vi "Kugel V9.vi"() -> ()   [LabVIEW 2020]
doc: "Illustrates the different data types that can be wired to the Case Selector terminal of a Case Structure. A Case Selector terminal can accept one of five possible data types: Boolean, error cluster, integer, enum, or string."
uses:
  Program Files (x86)/National Instruments/LabVIEW 2020/examples/Structures/Case Structure/support/Case Structure - Enum Options.ctl
  <vilib>/Utility/error.llb/DialogType.ctl
  <vilib>/DAQmx/write.llb/DAQmx Write (Digital Bool 1Line 1Point).vi
  <vilib>/DAQmx/read.llb/DAQmx Read (Analog DBL 1Chan 1Samp).vi
  <vilib>/Analysis/baseanly.llb/Mean (DBL).vi
  <vilib>/DAQmx/read.llb/DAQmx Read (Analog Wfm 1Chan NSamp).vi
  <vilib>/DAQmx/read.llb/DAQmx Read (Analog 1D Wfm NChan NSamp).vi
  <vilib>/DAQmx/create/channels.llb/DAQmx Create Channel (DO-Digital Output).vi
  <vilib>/DAQmx/create/channels.llb/DAQmx Create Channel (AI-Voltage-Basic).vi
  <vilib>/DAQmx/configure/timing.llb/DAQmx Timing (Sample Clock).vi
  <vilib>/DAQmx/miscellaneous.llb/DAQmx Fill In Error Info.vi
  <vilib>/DAQmx/configure/task.llb/DAQmx Configure Logging (TDMS).vi
  <vilib>/Waveform/WDTOps.llb/WDT Index Channel DBL.vi
  <vilib>/Analysis/NI_AALBase.lvlib
panel:
  out "P-Ex3 Max ungefilter":dbl caption="bar (max)" format="%0.2f"
  out "P-Ex3 Max gefilter":dbl caption="bar (max)" format="%0.2f"
  out "Current Save Path":path
  in  "User":string="unknown"
  in  "Serie":i32=1
  in  "Gas in Vol-%":dbl format="%.1f"
  in  "Gas":string(combo)="NoGas"
  in  "Weight [g]":dbl format="%.1f"
  in  "Dust":string(combo)="NoDust"
  out "Waveform Graph Staub":waveform(dbl)(graph)
  out "Pressure in V":dbl format="%0.3f"
  out "P-Ex3":dynamicdata(graph)
  out "P-Ex1":dynamicdata(graph)
  out "gemessene Spannungen":waveform(dbl)[](graph)
  in  "Ignition":bool
  in  "IN":bool
  in  "Reset":bool
  in  "OUT":bool
  in  "stop":bool
  out "Pressure in bar":dbl format="%0.3f"
  out "Pressure in bar":dbl(knob) scale=0.0..22.0
  in  "Option 1: manual operation\nOption 2: Ignition":T1
  # "Option 1"
  # "Option 2"
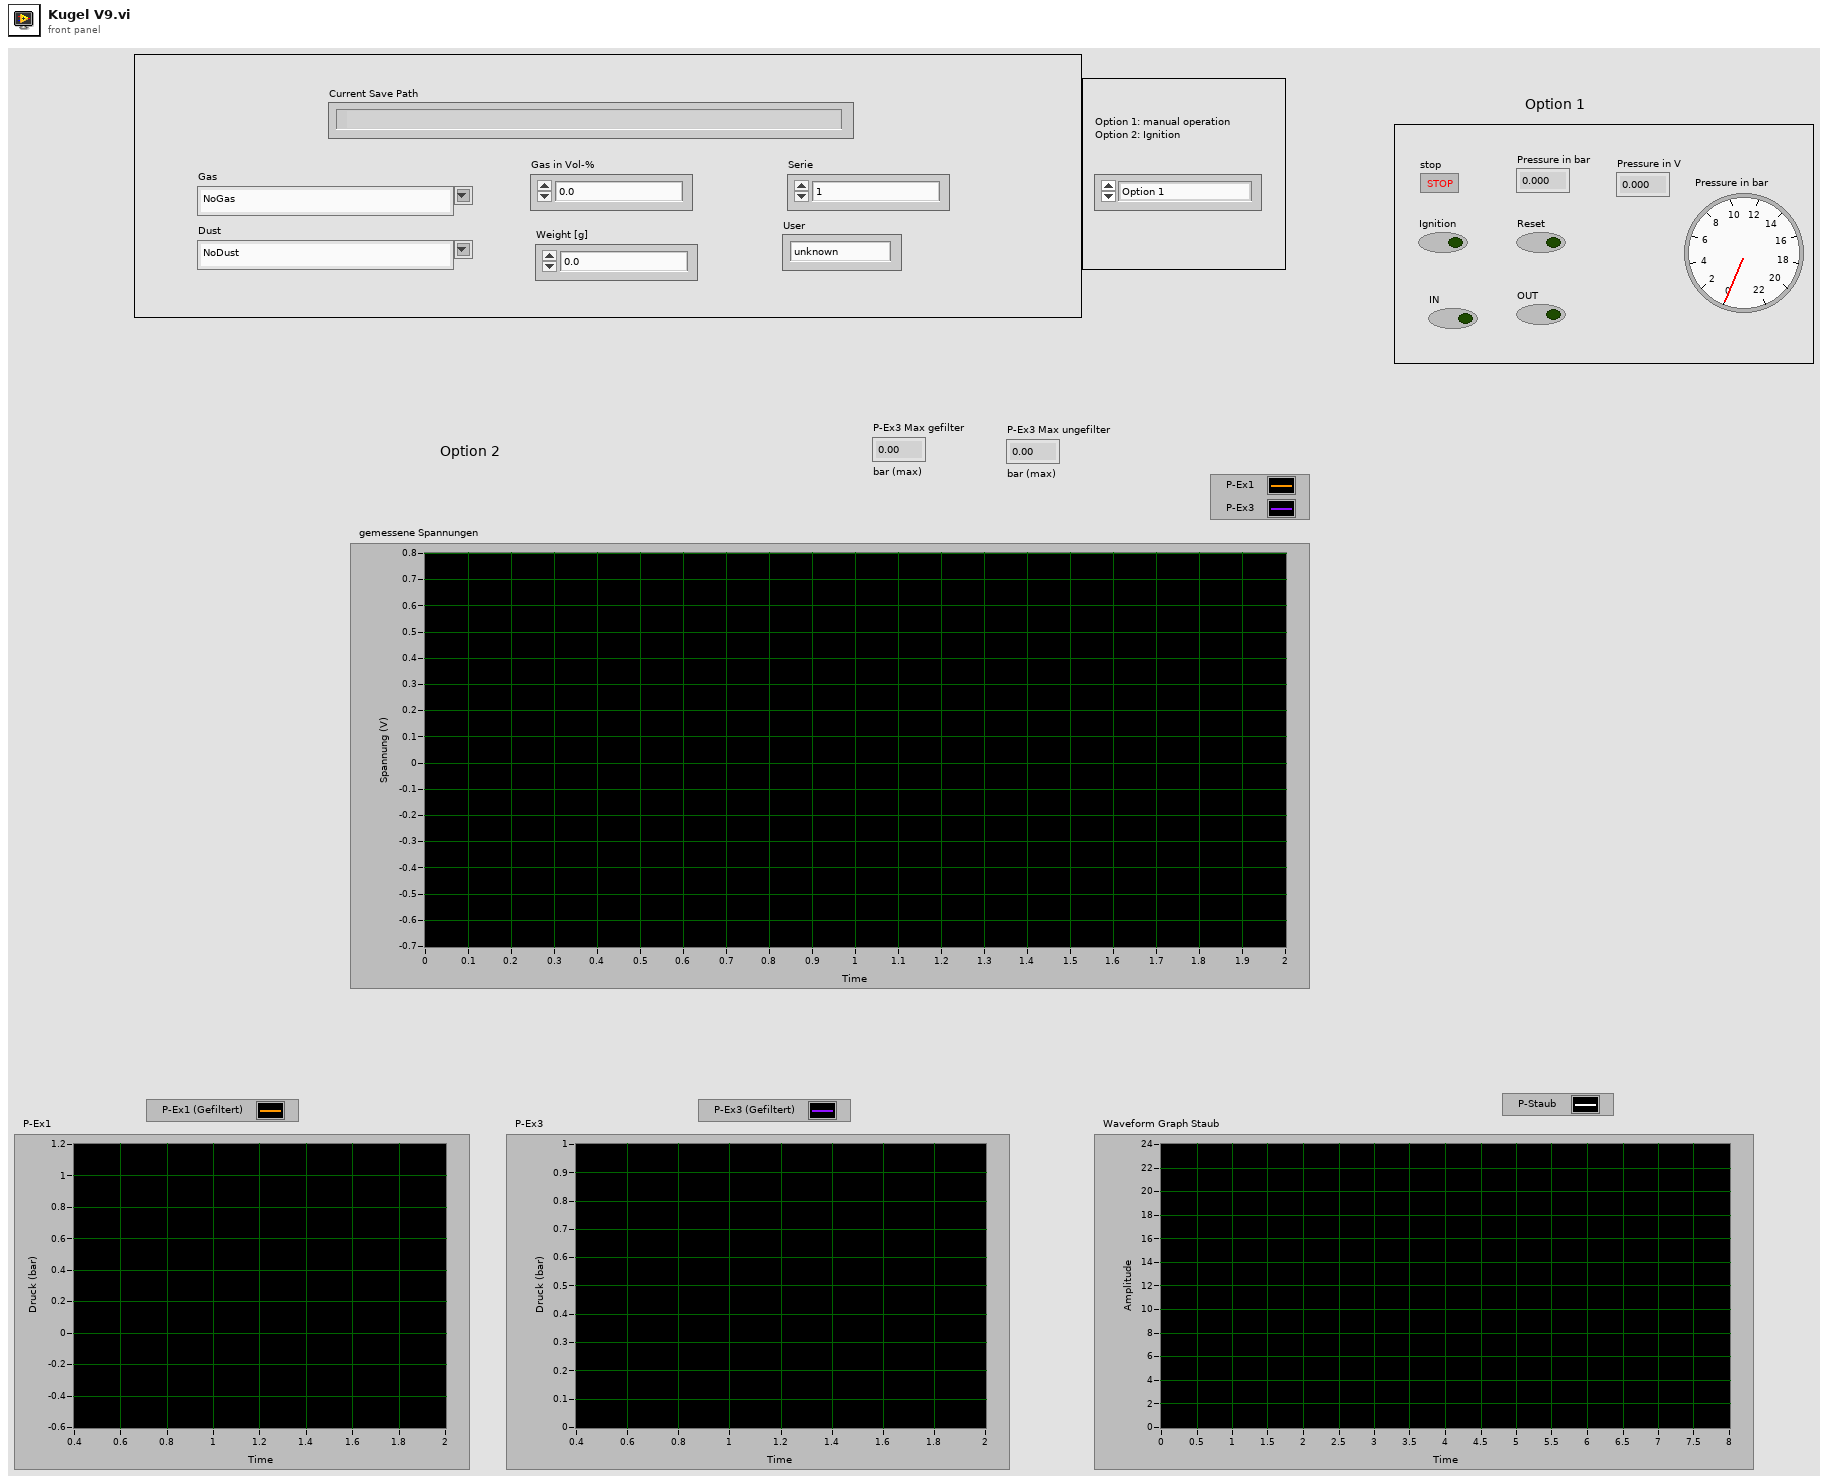
[diagram p1: front panel]
types:
  T1 = typedef "Case Structure - Enum Options.ctl" = enum16{"Option 1", "Option 2", "Option 3", "Option 4", "Option 5"}
  T2 = typedef "DialogType.ctl" = u16
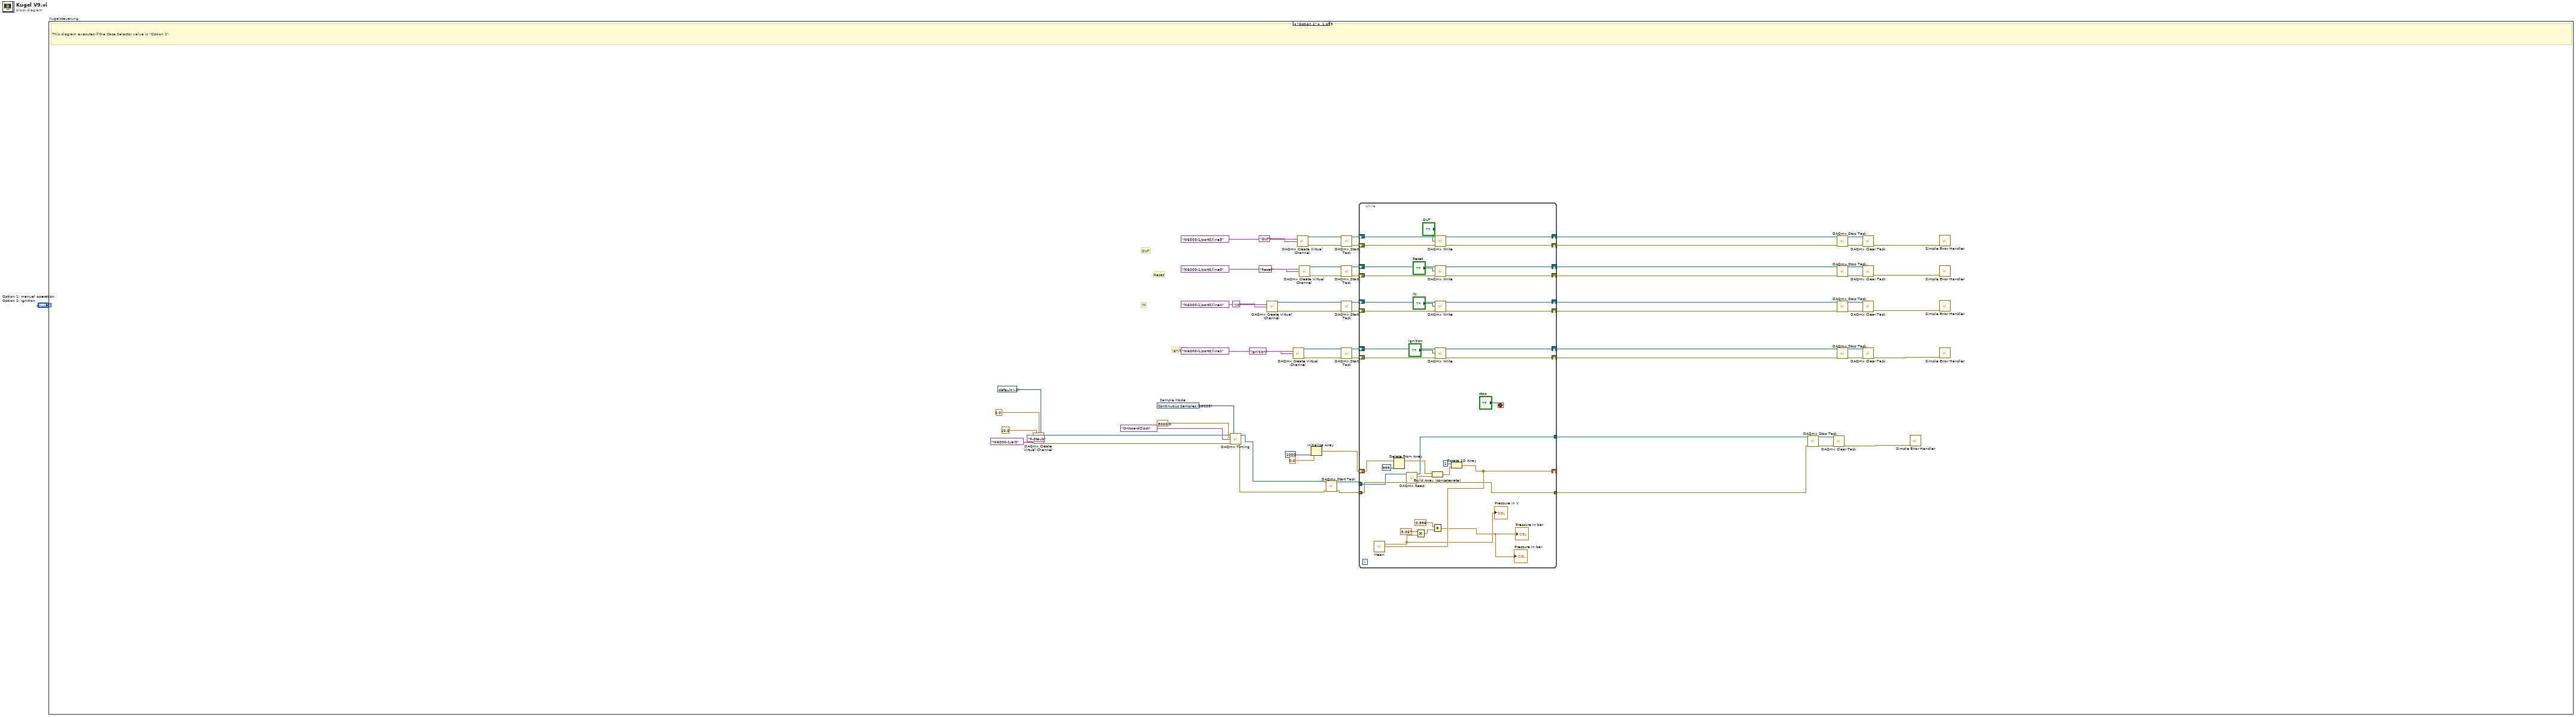
[diagram p0: block diagram]
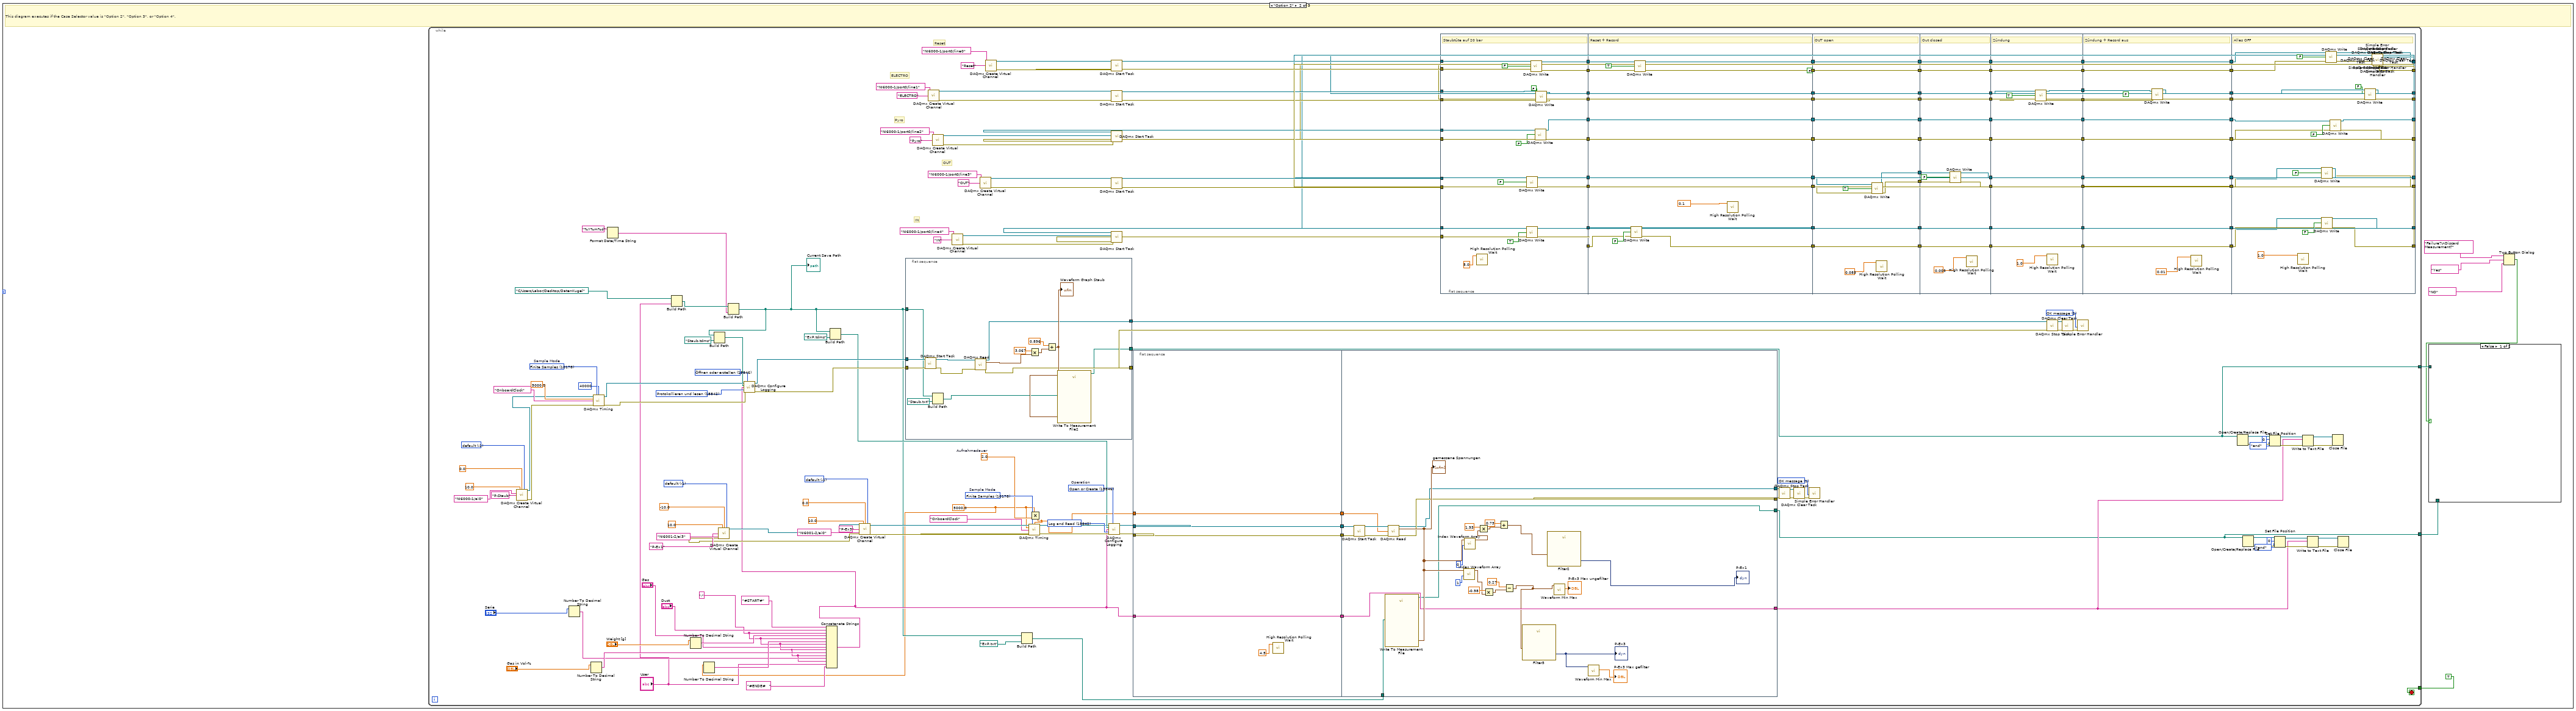
[diagram p2: hidden frame]
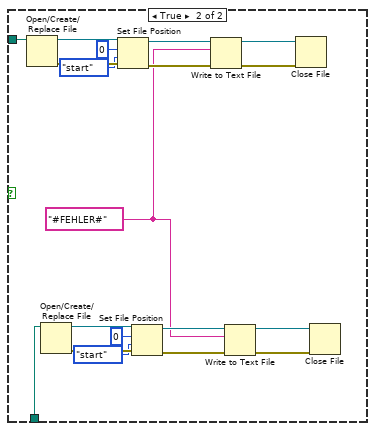
[diagram p3: hidden frame]
diagram:
  n1 = case "Kugelsteuerung" shown="\"Option 1\"" "Option 1: manual operation\nOption 2: Ignition" {
    frame "Option 1" {
      w19 = -1 items=["default"=-1, "RSE"=10083, "NRSE"=10078, "Differential"=10106, "Pseudodifferential"=12529] ("Terminal Configuration")
      w23 = 10123 items=["Finite Samples"=10178, "Continuous Samples"=10123, "Hardware Timed Single Point"=12522]  # Sample Mode
      # "Ignition"
      # "IN"
      # "OUT"
      # "Reset"
      # "This diagram executes if the Case Selector value is \"Option 1\"."
      n2 = call-poly <vilib>:"DAQmx Create Virtual Channel.vi"("maximum value"=10.0 ("Max Voltage P-Ex3"), "minimum value"=0.0 ("Min Voltage P-Ex3"), "input terminal configuration"=w19, "physical channels"=tag "NI6000-1/ai0" ("Physical Channel"), "name to assign"="P-Staub") -> ("task out"=w21:refnum<k21>, "error out"=w22:errorcluster)  [unwired: 9 in]
      n3 = call-poly <vilib>:"DAQmx Timing.vi"("task/channels in"=w21, "sample mode"=w23, "rate"=5000.0 ("Sample Rate"), "source"=tag "OnboardClock" ("Sample Clock Source"), "error in"=w22) -> ("task out"=w6:refnum<k21>, "error out"=w5:errorcluster)  [unwired: 9 in]
      n4 = call-poly <vilib>:"DAQmx Create Virtual Channel.vi"("lines"=tag "NI6000-1/port0/line4", "name to assign"="IN") -> ("task out"=w54:refnum<k21>, "error out"=w53:errorcluster)  [unwired: 12 in]
      n5 = call-poly <vilib>:"DAQmx Create Virtual Channel.vi"("lines"=tag "NI6000-1/port0/line1", "name to assign"="Ignition") -> ("task out"=w51:refnum<k21>, "error out"=w50:errorcluster)  [unwired: 12 in]
      n6 = call-poly <vilib>:"DAQmx Create Virtual Channel.vi"("lines"=tag "NI6000-1/port0/line3", "name to assign"="OUT") -> ("task out"=w57:refnum<k21>, "error out"=w56:errorcluster)  [unwired: 12 in]
      n7 = call-poly <vilib>:"DAQmx Create Virtual Channel.vi"("lines"=tag "NI6000-1/port0/line0", "name to assign"="Reset") -> ("task out"=w67:refnum<k21>, "error out"=w66:errorcluster)  [unwired: 12 in]
      n8 = Initialize Array(0.0 ("element"), 1000 ("dimension size")) -> (w4:dbl[])
      n9 = call <vilib>:"DAQmx Start Task.vi"("task/channels in"=w6, "error in"=w5) -> ("task out"=w8:refnum<k21>, "error out"=w7:errorcluster)  [unwired: 12 in]
      n10 = call <vilib>:"DAQmx Start Task.vi"("task/channels in"=w57, "error in"=w56) -> ("task out"=w29:refnum<k21>, "error out"=w28:errorcluster)  [unwired: 12 in]
      n11 = call <vilib>:"DAQmx Start Task.vi"("task/channels in"=w67, "error in"=w66) -> ("task out"=w31:refnum<k21>, "error out"=w30:errorcluster)  [unwired: 12 in]
      n12 = call <vilib>:"DAQmx Start Task.vi"("task/channels in"=w54, "error in"=w53) -> ("task out"=w25:refnum<k21>, "error out"=w24:errorcluster)  [unwired: 12 in]
      n13 = call <vilib>:"DAQmx Start Task.vi"("task/channels in"=w51, "error in"=w50) -> ("task out"=w27:refnum<k21>, "error out"=w26:errorcluster)  [unwired: 12 in]
      n14 = while {
        shift-right: [w104] -> w39
        shift-left: w31 -> [w96]
        shift-right: [w103] -> w38
        shift-left: w30 -> [w95]
        shift-right: [w102] -> w37
        shift-left: w29 -> [w94]
        shift-right: [w101] -> w36
        shift-left: w28 -> [w93]
        shift-right: [w100] -> w35
        shift-left: w27 -> [w92]
        shift-right: [w99] -> w34
        shift-left: w26 -> [w91]
        shift-right: [w98] -> w33
        shift-left: w25 -> [w90]
        shift-right: [w97] -> w32
        shift-left: w24 -> [w89]
        tunnel: w8 -> [w83]
        tunnel: w7 -> [w82]
        tunnel: [w81] -> w11
        tunnel: [w80] -> w10
        shift-right: [w74] -> _
        shift-left: w4 -> [w78]
        stop <- "stop" stop-if-true
        n15 = Delete From Array(array=w78, index=999) -> (array with subset deleted=w77:dbl[])  [unwired: 1 in, 1 out]
        n16 = call-poly <vilib>:"DAQmx Read.vi"("task/channels in"=w83, "error in"=w82) -> ("task out"=w81:refnum<k21>, "data"=w79:dbl, "error out"=w80:errorcluster)  [unwired: 11 in]
        n17 = Build Array (concatenate)(w77, w79) -> (w75:dbl[])
        n18 = call-poly <vilib>:"DAQmx Write.vi"("task/channels in"=w94, "data"="OUT", "error in"=w93) -> ("task out"=w102:refnum<k21>, "error out"=w101:errorcluster)  [unwired: 10 in, 1 out]
        n19 = call-poly <vilib>:"DAQmx Write.vi"("task/channels in"=w96, "data"="Reset", "error in"=w95) -> ("task out"=w104:refnum<k21>, "error out"=w103:errorcluster)  [unwired: 10 in, 1 out]
        n20 = call-poly <vilib>:"DAQmx Write.vi"("task/channels in"=w90, "data"="IN", "error in"=w89) -> ("task out"=w98:refnum<k21>, "error out"=w97:errorcluster)  [unwired: 10 in, 1 out]
        n21 = call-poly <vilib>:"DAQmx Write.vi"("task/channels in"=w92, "data"="Ignition", "error in"=w91) -> ("task out"=w100:refnum<k21>, "error out"=w99:errorcluster)  [unwired: 10 in, 1 out]
        n22 = Rotate 1D Array(1:w75, 2:1 ("n")) -> (0:w74:dbl[])
        n23 = call-poly <vilib>:"Mean.vi"("X"=w74) -> ("mean"=w68:dbl)  [unwired: 1 out]
        "Pressure in V" <- w68
        n24 = Multiply(x=3.067, y=w68) -> (x*y=w72:dbl)
        n25 = Add(x=0.896 ("y"), y=w72) -> (x+y=→"Pressure in bar" →"Pressure in bar":dbl)
      }
      n26 = call <vilib>:"DAQmx Stop Task.vi"("task/channels in"=w11, "error in"=w10) -> ("task out"=w14:refnum<k21>, "error out"=w13:errorcluster)  [unwired: 12 in]
      n27 = call <vilib>:"DAQmx Clear Task.vi"("task in"=w14, "error in"=w13) -> ("error out"=w12:errorcluster)  [unwired: 13 in]
      n28 = call <vilib>:"DAQmx Stop Task.vi"("task/channels in"=w37, "error in"=w36) -> ("task out"=w61:refnum<k21>, "error out"=w60:errorcluster)  [unwired: 12 in]
      n29 = call <vilib>:"DAQmx Stop Task.vi"("task/channels in"=w39, "error in"=w38) -> ("task out"=w65:refnum<k21>, "error out"=w64:errorcluster)  [unwired: 12 in]
      n30 = call <vilib>:"DAQmx Stop Task.vi"("task/channels in"=w33, "error in"=w32) -> ("task out"=w46:refnum<k21>, "error out"=w45:errorcluster)  [unwired: 12 in]
      n31 = call <vilib>:"DAQmx Stop Task.vi"("task/channels in"=w35, "error in"=w34) -> ("task out"=w49:refnum<k21>, "error out"=w48:errorcluster)  [unwired: 12 in]
      n32 = call <vilib>:"DAQmx Clear Task.vi"("task in"=w61, "error in"=w60) -> ("error out"=w59:errorcluster)  [unwired: 13 in]
      n33 = call <vilib>:"DAQmx Clear Task.vi"("task in"=w65, "error in"=w64) -> ("error out"=w63:errorcluster)  [unwired: 13 in]
      n34 = call <vilib>:"DAQmx Clear Task.vi"("task in"=w46, "error in"=w45) -> ("error out"=w44:errorcluster)  [unwired: 13 in]
      n35 = call <vilib>:"DAQmx Clear Task.vi"("task in"=w49, "error in"=w48) -> ("error out"=w47:errorcluster)  [unwired: 13 in]
      n36 = call <vilib>:"Simple Error Handler.vi"("error in (no error)"=w12) -> ()  [unwired: 4 in, 5 out]
      n37 = call <vilib>:"Simple Error Handler.vi"("error in (no error)"=w59) -> ()  [unwired: 4 in, 5 out]
      n38 = call <vilib>:"Simple Error Handler.vi"("error in (no error)"=w63) -> ()  [unwired: 4 in, 5 out]
      n39 = call <vilib>:"Simple Error Handler.vi"("error in (no error)"=w44) -> ()  [unwired: 4 in, 5 out]
      n40 = call <vilib>:"Simple Error Handler.vi"("error in (no error)"=w47) -> ()  [unwired: 4 in, 5 out]
    }
    frame "Option 2" {
      # "This diagram executes if the Case Selector value is \"Option 2\", \"Option 3\", or \"Option 4\"."
      n41 = while {
        tunnel: TRUE ("Stopp-Schaltfläche") -> [w201]
        tunnel: [w145] -> w110
        tunnel: [w144] -> w109
        stop <- w201 stop-if-true
        w131 = 5000.0 ("Sample Rate")
        w165 = ";" ("String")
        w180 = 15846 items=["Öffnen"=10437, "Öffnen oder erstellen"=15846, "Erstellen oder ersetzen"=15847, "Erstellen"=15848] ("operation")
        w181 = 15842 items=["Aus"=10231, "Protokoll"=15844, "Protokollieren und lesen"=15842] ("logging mode")
        w189 = -1 items=["default"=-1, "RSE"=10083, "NRSE"=10078, "Differential"=10106, "Pseudodifferential"=12529] ("Terminal Configuration")
        w194 = 10178 items=["Finite Samples"=10178, "Continuous Samples"=10123, "Hardware Timed Single Point"=12522]  # Sample Mode
        w197 = T2 1 items=["no dialog", "OK message", "continue or stop message", "OK message + warnings", "continue/stop + warnings"] ("type of dialog (OK msg:1)")
        w208 = 2.0  # Aufnahmedauer
        w210 = T2 1 items=["no dialog", "OK message", "continue or stop message", "OK message + warnings", "continue/stop + warnings"] ("type of dialog (OK msg:1)")
        w226 = 15842 items=["Off"=10231, "Log and Read"=15842] ("Logging Mode")
        w224 = -1 items=["default"=-1, "RSE"=10083, "NRSE"=10078, "Differential"=10106, "Pseudodifferential"=12529] ("Terminal Configuration")
        w216 = -1 items=["default"=-1, "RSE"=10083, "NRSE"=10078, "Differential"=10106, "Pseudodifferential"=12529] ("Terminal Configuration 3")
        w227 = 15846 items=["Open"=10437, "Open or Create"=15846, "Create or Replace"=15847, "Create"=15848]  # Operation
        w230 = 10178 items=["Finite Samples"=10178, "Continuous Samples"=10123, "Hardware Timed Single Point"=12522]  # Sample Mode
        # "ELECTRO"
        # "Pyro"
        # "IN"
        # "OUT"
        # "Reset"
        n42 = call-poly <vilib>:"DAQmx Create Virtual Channel.vi"("maximum value"=10.0 ("Max Voltage P-Ex3"), "minimum value"=0.0 ("Min Voltage P-Ex3"), "input terminal configuration"=w189, "physical channels"=tag "NI6000-1/ai0" ("Physical Channel"), "name to assign"="P-Staub") -> ("task out"=w185:refnum<k21>, "error out"=w186:errorcluster)  [unwired: 9 in]
        n43 = Number To Decimal String(number="Serie") -> (decimal integer string=w166:string)  [unwired: 1 in]
        n44 = Number To Decimal String(number="Gas in Vol-%") -> (decimal integer string=w168:string)  [unwired: 1 in]
        n45 = call-poly <vilib>:"DAQmx Timing.vi"("task/channels in"=w185, "sample mode"=w194, "samples per channel"=40000, "rate"=5000.0 ("Sample Rate"), "source"=tag "OnboardClock" ("Sample Clock Source"), "error in"=w186) -> ("task out"=w183:refnum<k21>, "error out"=w182:errorcluster)  [unwired: 8 in]
        n46 = Format Date/Time String(time format string (%c)="%Y%m%d" ("Zeitformatierungs-String (%c)")) -> (date/time string=w140:string)  [unwired: 2 in]
        n47 = Build Path(base path=path "C:/Users/Labor/Desktop/DatenKugel" ("Choose Path"), name or relative path="User") -> (appended path=w142:path)
        n48 = Number To Decimal String(number="Weight [g]") -> (decimal integer string=w173:string)  [unwired: 1 in]
        n49 = Number To Decimal String(number=w131) -> (decimal integer string=w171:string)  [unwired: 1 in]
        n50 = call-poly <vilib>:"DAQmx Create Virtual Channel.vi"("maximum value"=10.0 ("Max Voltage P-Ex1"), "minimum value"=-10.0 ("Min Voltage P-Ex1"), "input terminal configuration"=w216, "physical channels"=tag "NI6001-2/ai3" ("Physical Channel 3"), "name to assign"="P-Ex1") -> ("task out"=w203:refnum<k21>, "error out"=w202:errorcluster)  [unwired: 9 in]
        n51 = Build Path(base path=w142, name or relative path=w140) -> (appended path=w133:path)
        "Current Save Path" <- w133
        n52 = Build Path(base path=w133, name or relative path=path "Staub.tdms" ("Name oder relativer Pfad")) -> (appended path=w138:path)
        n53 = Concatenate Strings("#START#" ("String"), "Dust", w165, w173, w165, w171, w165, "Gas", w165, w168, w165, w166, w165, "User", "#ENDE#   " ("String")) -> (w175:string)
        n54 = call-poly <vilib>:"DAQmx Configure Logging.vi"("task/channels in"=w183, "operation"=w180, "file path"=w138, "group name"=w175, "logging mode"=w181, "error in"=w182) -> ("task out"=w179:refnum<k21>, "error out"=w178:errorcluster)  [unwired: 8 in]
        n55 = Build Path(base path=w133, name or relative path=path "ExP.tdms" ("Name oder relativer Pfad")) -> (appended path=w134:path)
        n56 = call-poly <vilib>:"DAQmx Create Virtual Channel.vi"("task in"=w203, "maximum value"=10.0 ("Max Voltage P-Ex3"), "minimum value"=0.0 ("Min Voltage P-Ex3"), "input terminal configuration"=w224, "physical channels"=tag "NI6001-2/ai0" ("Physical Channel"), "name to assign"="P-Ex3", "error in"=w202) -> ("task out"=w228:refnum<k21>, "error out"=w229:errorcluster)  [unwired: 7 in]
        n57 = flat-sequence {
          tunnel: w179 -> [w359]
          tunnel: w178 -> [w358]
          tunnel: [w354] -> w177
          tunnel: [w353] -> w176
          tunnel: [w352] -> w145
          tunnel: w133 -> [w351]
          frame #0 {
            n58 = call <vilib>:"DAQmx Start Task.vi"("task/channels in"=w359, "error in"=w358) -> ("task out"=w362:refnum<k21>, "error out"=w363:errorcluster)  [unwired: 12 in]
            n59 = Build Path(base path=w351, name or relative path=path "Staub.txt" ("Name oder relativer Pfad")) -> (appended path=w349:path)
            n60 = call-poly <vilib>:"DAQmx Read.vi"("task/channels in"=w362, "error in"=w363) -> ("task out"=w354:refnum<k21>, "data"=w361:waveform(dbl), "error out"=w353:errorcluster)  [unwired: 11 in]
            n61 = Multiply(x=3.067, y=w361) -> (x*y=w360:waveform(dbl))
            n62 = Add(x=0.896 ("y"), y=w360) -> (x+y=w355:waveform(dbl))
            "Waveform Graph Staub" <- w355
            n63 = call "Write To Measurement File2"("Signals"=w355, "Filename"=w349) -> ("Filename Out"=w352:path)  [unwired: 15 in, 2 out]
          }
        }
        n64 = call-poly <vilib>:"DAQmx Create Virtual Channel.vi"("lines"=tag "NI6000-1/port0/line1", "name to assign"="ELECTRO") -> ("task out"=w258:refnum<k21>, "error out"=w257:errorcluster)  [unwired: 12 in]
        n65 = call-poly <vilib>:"DAQmx Create Virtual Channel.vi"("lines"=tag "NI6000-1/port0/line2", "name to assign"="Pyro") -> ("task out"=w261:refnum<k21>, "error out"=w260:errorcluster)  [unwired: 12 in]
        n66 = call-poly <vilib>:"DAQmx Create Virtual Channel.vi"("lines"=tag "NI6000-1/port0/line4", "name to assign"="IN") -> ("task out"=w264:refnum<k21>, "error out"=w263:errorcluster)  [unwired: 12 in]
        n67 = call-poly <vilib>:"DAQmx Create Virtual Channel.vi"("lines"=tag "NI6000-1/port0/line3", "name to assign"="OUT") -> ("task out"=w271:refnum<k21>, "error out"=w269:errorcluster)  [unwired: 12 in]
        n68 = call-poly <vilib>:"DAQmx Create Virtual Channel.vi"("lines"=tag "NI6000-1/port0/line0", "name to assign"="Reset") -> ("task out"=w284:refnum<k21>, "error out"=w283:errorcluster)  [unwired: 12 in]
        n69 = Build Path(base path=w133, name or relative path=path "ExP.txt" ("Name oder relativer Pfad")) -> (appended path=w136:path)
        n70 = Multiply(x=w131, y=w208) -> (x*y=w195:dbl)
        n71 = call-poly <vilib>:"DAQmx Timing.vi"("task/channels in"=w228, "sample mode"=w230, "samples per channel"=w195, "rate"=w131, "source"=tag "OnboardClock" ("Sample Clock Source"), "error in"=w229) -> ("task out"=w220:refnum<k21>, "error out"=w219:errorcluster)  [unwired: 8 in]
        n72 = call-poly <vilib>:"DAQmx Configure Logging.vi"("task/channels in"=w220, "operation"=w227, "file path"=w134, "group name"=w175, "logging mode"=w226, "error in"=w219) -> ("task out"=w205:refnum<k21>, "error out"=w204:errorcluster)  [unwired: 8 in]
        n73 = call <vilib>:"DAQmx Start Task.vi"("task/channels in"=w284, "error in"=w283) -> ("task out"=w285:refnum<k21>, "error out"=w282:errorcluster)  [unwired: 12 in]
        n74 = call <vilib>:"DAQmx Start Task.vi"("task/channels in"=w258, "error in"=w257) -> ("task out"=w256:refnum<k21>, "error out"=w255:errorcluster)  [unwired: 12 in]
        n75 = call <vilib>:"DAQmx Start Task.vi"("task/channels in"=w261, "error in"=w260) -> ("task out"=w254:refnum<k21>, "error out"=w253:errorcluster)  [unwired: 12 in]
        n76 = call <vilib>:"DAQmx Start Task.vi"("task/channels in"=w271, "error in"=w269) -> ("task out"=w270:refnum<k21>, "error out"=w268:errorcluster)  [unwired: 12 in]
        n77 = call <vilib>:"DAQmx Start Task.vi"("task/channels in"=w264, "error in"=w263) -> ("task out"=w252:refnum<k21>, "error out"=w251:errorcluster)  [unwired: 12 in]
        n78 = flat-sequence {
          tunnel: w204 -> [w367]
          tunnel: w205 -> [w368]
          tunnel: w175 -> [w364]
          tunnel: [w364] -> w288
          tunnel: [w368] -> w287
          tunnel: [w367] -> w286
          tunnel: w195 -> [w365]
          tunnel: [w365] -> w196
          tunnel: [w378] -> w207
          tunnel: [w379] -> w206
          tunnel: w288 -> [w377]
          tunnel: w287 -> [w395]
          tunnel: w286 -> [w394]
          tunnel: w196 -> [w380]
          tunnel: [w376] -> w144
          tunnel: [w377] -> w150
          tunnel: w136 -> [w375]
          frame #0 {
            n79 = call <vilib>:"High Resolution Polling Wait.vi"("seconds to wait"=4.5 ("Staubtüte füllen")) -> ()  [unwired: 10 in, 1 out]
          }
          frame #1 {
            n80 = call <vilib>:"DAQmx Start Task.vi"("task/channels in"=w395, "error in"=w394) -> ("task out"=w392:refnum<k21>, "error out"=w393:errorcluster)  [unwired: 12 in]
            n81 = call-poly <vilib>:"DAQmx Read.vi"("task/channels in"=w392, "number of samples per channel"=w380, "error in"=w393) -> ("task out"=w378:refnum<k21>, "data"=w382:waveform(dbl)[], "error out"=w379:errorcluster)  [unwired: 10 in]
            "gemessene Spannungen" <- w382
            n82 = call "Write To Measurement File"("Signals"=w382, "Filename"=w375) -> ("Filename Out"=w376:path)  [unwired: 15 in, 2 out]
            n83 = call-poly <vilib>:"Index Waveform Array.vi"("index"=1, "waveform array"=w382) -> ("waveform"=w381:waveform(dbl))  [unwired: 8 in, 1 out]
            n84 = call-poly <vilib>:"Index Waveform Array.vi"("index"=0, "waveform array"=w382) -> ("waveform"=w383:waveform(dbl))  [unwired: 8 in, 1 out]
            n85 = Multiply(x=1.93, y=w383) -> (x*y=w385:waveform(dbl))
            n86 = Multiply(x=-0.98, y=w381) -> (x*y=w388:waveform(dbl))
            n87 = Add(x=0.73, y=w385) -> (x+y=w374:waveform(dbl))
            n88 = Subtract(x=0.27, y=w388) -> (x-y=w370:waveform(dbl))
            n89 = call "Filter3"("Signal"=w370) -> ("Filtered Signal"=w372:dynamicdata)  [unwired: 9 in, 1 out]
            "P-Ex3" <- w372
            n90 = call "Filter2"("Signal"=w374) -> ("Filtered Signal"=→"P-Ex1":dynamicdata)  [unwired: 9 in, 1 out]
            n91 = call <vilib>:"Waveform Min Max.vi"("waveform in"=w370) -> ("Y max"=→"P-Ex3 Max ungefilter":dbl)  [unwired: 5 in, 5 out]
            n92 = call <vilib>:"Waveform Min Max.vi"("waveform in"=w372) -> ("Y max"=→"P-Ex3 Max gefilter":dbl)  [unwired: 5 in, 5 out]
          }
        }
        n93 = flat-sequence {
          tunnel: w285 -> [w419]
          tunnel: w282 -> [w418]
          tunnel: w270 -> [w417]
          tunnel: w268 -> [w415]
          tunnel: w256 -> [w413]
          tunnel: w255 -> [w412]
          tunnel: w254 -> [w411]
          tunnel: w253 -> [w410]
          tunnel: w252 -> [w409]
          tunnel: w251 -> [w408]
          tunnel: [w421] -> w348
          tunnel: [w420] -> w347
          tunnel: [w416] -> w346
          tunnel: [w414] -> w345
          tunnel: [w407] -> w344
          tunnel: [w406] -> w343
          tunnel: [w405] -> w342
          tunnel: [w404] -> w341
          tunnel: [w403] -> w340
          tunnel: [w402] -> w339
          tunnel: w348 -> [w430]
          tunnel: w347 -> [w431]
          tunnel: w346 -> [w438]
          tunnel: w345 -> [w437]
          tunnel: w344 -> [w436]
          tunnel: w343 -> [w435]
          tunnel: w342 -> [w434]
          tunnel: w341 -> [w433]
          tunnel: w340 -> [w425]
          tunnel: w339 -> [w424]
          tunnel: [w429] -> w338
          tunnel: [w428] -> w337
          tunnel: [w438] -> w336
          tunnel: [w437] -> w335
          tunnel: [w436] -> w334
          tunnel: [w435] -> w333
          tunnel: [w434] -> w332
          tunnel: [w433] -> w331
          tunnel: [w422] -> w330
          tunnel: [w423] -> w329
          tunnel: w338 -> [w440]
          tunnel: w337 -> [w439]
          tunnel: w336 -> [w444]
          tunnel: w335 -> [w443]
          tunnel: w334 -> [w452]
          tunnel: w333 -> [w451]
          tunnel: w332 -> [w450]
          tunnel: w331 -> [w449]
          tunnel: w330 -> [w448]
          tunnel: w329 -> [w447]
          tunnel: [w439] -> w328
          tunnel: [w452] -> w327
          tunnel: [w451] -> w326
          tunnel: [w450] -> w325
          tunnel: [w449] -> w324
          tunnel: [w448] -> w323
          tunnel: [w447] -> w322
          tunnel: [w442] -> w321
          tunnel: [w441] -> w320
          tunnel: [w440] -> w319
          tunnel: w328 -> [w465]
          tunnel: w327 -> [w464]
          tunnel: w326 -> [w463]
          tunnel: w325 -> [w462]
          tunnel: w324 -> [w461]
          tunnel: w323 -> [w460]
          tunnel: w322 -> [w459]
          tunnel: [w466] -> w318
          tunnel: [w465] -> w317
          tunnel: [w456] -> w316
          tunnel: [w464] -> w315
          tunnel: [w463] -> w314
          tunnel: [w462] -> w313
          tunnel: [w461] -> w312
          tunnel: [w460] -> w311
          tunnel: [w459] -> w310
          tunnel: w321 -> [w457]
          tunnel: [w455] -> w309
          tunnel: w320 -> [w454]
          tunnel: w319 -> [w466]
          tunnel: w318 -> [w480]
          tunnel: w317 -> [w479]
          tunnel: w316 -> [w477]
          tunnel: w315 -> [w470]
          tunnel: w314 -> [w469]
          tunnel: w313 -> [w471]
          tunnel: w312 -> [w472]
          tunnel: w311 -> [w476]
          tunnel: w310 -> [w475]
          tunnel: [w480] -> w308
          tunnel: [w479] -> w307
          tunnel: [w478] -> w306
          tunnel: [w477] -> w305
          tunnel: [w476] -> w304
          tunnel: [w475] -> w303
          tunnel: w309 -> [w478]
          tunnel: [w472] -> w302
          tunnel: [w471] -> w301
          tunnel: [w468] -> w300
          tunnel: [w467] -> w299
          tunnel: w308 -> [w494]
          tunnel: w307 -> [w493]
          tunnel: w306 -> [w492]
          tunnel: w305 -> [w491]
          tunnel: w304 -> [w490]
          tunnel: w303 -> [w489]
          tunnel: [w494] -> w298
          tunnel: [w493] -> w297
          tunnel: [w492] -> w296
          tunnel: [w491] -> w295
          tunnel: [w482] -> w294
          tunnel: [w490] -> w293
          tunnel: [w489] -> w292
          tunnel: [w486] -> w291
          tunnel: [w485] -> w290
          tunnel: w302 -> [w486]
          tunnel: w301 -> [w485]
          tunnel: w300 -> [w484]
          tunnel: w299 -> [w483]
          tunnel: [w481] -> w289
          tunnel: [w495] -> w236
          tunnel: [w496] -> w237
          tunnel: [w499] -> w238
          tunnel: [w500] -> w239
          tunnel: [w501] -> w240
          tunnel: [w502] -> w241
          tunnel: [w497] -> w267
          tunnel: [w498] -> w266
          tunnel: [w503] -> w277
          tunnel: [w514] -> w281
          tunnel: w298 -> [w515]
          tunnel: w297 -> [w513]
          tunnel: w296 -> [w507]
          tunnel: w295 -> [w510]
          tunnel: w294 -> [w505]
          tunnel: w293 -> [w508]
          tunnel: w292 -> [w509]
          tunnel: w291 -> [w511]
          tunnel: w290 -> [w506]
          tunnel: w289 -> [w512]
          frame #0 {
            # "Staubtüte auf 20 bar"
            n94 = call <vilib>:"High Resolution Polling Wait.vi"("seconds to wait"=5.0 ("Staubtüte füllen")) -> ()  [unwired: 10 in, 1 out]
            n95 = call-poly <vilib>:"DAQmx Write.vi"("task/channels in"=w409, "data"=TRUE ("IN"), "error in"=w408) -> ("task out"=w403:refnum<k21>, "error out"=w402:errorcluster)  [unwired: 10 in, 1 out]
            n96 = call-poly <vilib>:"DAQmx Write.vi"("task/channels in"=w417, "data"=FALSE ("OUT"), "error in"=w415) -> ("task out"=w416:refnum<k21>, "error out"=w414:errorcluster)  [unwired: 10 in, 1 out]
            n97 = call-poly <vilib>:"DAQmx Write.vi"("task/channels in"=w419, "data"=FALSE ("Reset"), "error in"=w418) -> ("task out"=w421:refnum<k21>, "error out"=w420:errorcluster)  [unwired: 10 in, 1 out]
            n98 = call-poly <vilib>:"DAQmx Write.vi"("task/channels in"=w411, "data"=FALSE ("Pyro"), "error in"=w410) -> ("task out"=w405:refnum<k21>, "error out"=w404:errorcluster)  [unwired: 10 in, 1 out]
            n99 = call-poly <vilib>:"DAQmx Write.vi"("task/channels in"=w413, "data"=FALSE ("ELECTRO"), "error in"=w412) -> ("task out"=w407:refnum<k21>, "error out"=w406:errorcluster)  [unwired: 10 in, 1 out]
          }
          frame #1 {
            # "Reset + Record"
            n100 = call-poly <vilib>:"DAQmx Write.vi"("task/channels in"=w425, "data"=FALSE ("IN"), "error in"=w424) -> ("task out"=w422:refnum<k21>, "error out"=w423:errorcluster)  [unwired: 10 in, 1 out]
            n101 = call-poly <vilib>:"DAQmx Write.vi"("task/channels in"=w430, "data"=TRUE ("Reset"), "error in"=w431) -> ("task out"=w429:refnum<k21>, "error out"=w428:errorcluster)  [unwired: 10 in, 1 out]
            n102 = call <vilib>:"High Resolution Polling Wait.vi"("seconds to wait"=0.1 ("Reset Record")) -> ()  [unwired: 10 in, 1 out]
          }
          frame #2 {
            (unwired) FALSE ("Reset")
            # "OUT open"
            n103 = call-poly <vilib>:"DAQmx Write.vi"("task/channels in"=w444, "data"=TRUE ("OUT"), "error in"=w443) -> ("task out"=w441:refnum<k21>, "error out"=w442:errorcluster)  [unwired: 10 in, 1 out]
            n104 = call <vilib>:"High Resolution Polling Wait.vi"("seconds to wait"=0.085 ("OUT open")) -> ()  [unwired: 10 in, 1 out]
          }
          frame #3 {
            # "Out closed"
            n105 = call-poly <vilib>:"DAQmx Write.vi"("task/channels in"=w454, "data"=FALSE ("OUT"), "error in"=w457) -> ("task out"=w455:refnum<k21>, "error out"=w456:errorcluster)  [unwired: 10 in, 1 out]
            n106 = call <vilib>:"High Resolution Polling Wait.vi"("seconds to wait"=0.005 ("OUT closed")) -> ()  [unwired: 10 in, 1 out]
          }
          frame #4 {
            # "Zündung"
            n107 = call-poly <vilib>:"DAQmx Write.vi"("task/channels in"=w470, "data"=TRUE ("OUT"), "error in"=w469) -> ("task out"=w467:refnum<k21>, "error out"=w468:errorcluster)  [unwired: 10 in, 1 out]
            n108 = call <vilib>:"High Resolution Polling Wait.vi"("seconds to wait"=1.0 ("Zündimpuls")) -> ()  [unwired: 10 in, 1 out]
          }
          frame #5 {
            # "Zündung + Record aus"
            n109 = call-poly <vilib>:"DAQmx Write.vi"("task/channels in"=w483, "data"=FALSE ("OUT"), "error in"=w484) -> ("task out"=w482:refnum<k21>, "error out"=w481:errorcluster)  [unwired: 10 in, 1 out]
            n110 = call <vilib>:"High Resolution Polling Wait.vi"("seconds to wait"=0.01 ("Zündung aus")) -> ()  [unwired: 10 in, 1 out]
          }
          frame #6 {
            # "Alles OFF"
            n111 = call <vilib>:"High Resolution Polling Wait.vi"("seconds to wait"=1.0 ("alles aus")) -> ()  [unwired: 10 in, 1 out]
            n112 = call-poly <vilib>:"DAQmx Write.vi"("task/channels in"=w508, "data"=FALSE ("IN"), "error in"=w509) -> ("task out"=w496:refnum<k21>, "error out"=w495:errorcluster)  [unwired: 10 in, 1 out]
            n113 = call-poly <vilib>:"DAQmx Write.vi"("task/channels in"=w507, "data"=FALSE ("OUT"), "error in"=w510) -> ("task out"=w498:refnum<k21>, "error out"=w497:errorcluster)  [unwired: 10 in, 1 out]
            n114 = call-poly <vilib>:"DAQmx Write.vi"("task/channels in"=w515, "data"=FALSE ("Reset"), "error in"=w513) -> ("task out"=w514:refnum<k21>, "error out"=w503:errorcluster)  [unwired: 10 in, 1 out]
            n115 = call-poly <vilib>:"DAQmx Write.vi"("task/channels in"=w506, "data"=FALSE ("Pyro"), "error in"=w511) -> ("task out"=w500:refnum<k21>, "error out"=w499:errorcluster)  [unwired: 10 in, 1 out]
            n116 = call-poly <vilib>:"DAQmx Write.vi"("task/channels in"=w505, "data"=FALSE, "error in"=w512) -> ("task out"=w502:refnum<k21>, "error out"=w501:errorcluster)  [unwired: 10 in, 1 out]
          }
        }
        n117 = call <vilib>:"DAQmx Stop Task.vi"("task/channels in"=w207, "error in"=w206) -> ("task out"=w211:refnum<k21>, "error out"=w212:errorcluster)  [unwired: 12 in]
        n118 = call <vilib>:"DAQmx Clear Task.vi"("task in"=w211, "error in"=w212) -> ("error out"=w209:errorcluster)  [unwired: 13 in]
        n119 = call <vilib>:"Simple Error Handler.vi"("type of dialog (OK msg:1)"=w210, "error in (no error)"=w209) -> ()  [unwired: 3 in, 5 out]
        n120 = call <vilib>:"DAQmx Stop Task.vi"("task/channels in"=w177, "error in"=w176) -> ("task out"=w199:refnum<k21>, "error out"=w198:errorcluster)  [unwired: 12 in]
        n121 = call <vilib>:"DAQmx Clear Task.vi"("task in"=w199, "error in"=w198) -> ("error out"=w200:errorcluster)  [unwired: 13 in]
        n122 = call <vilib>:"Simple Error Handler.vi"("type of dialog (OK msg:1)"=w197, "error in (no error)"=w200) -> ()  [unwired: 3 in, 5 out]
        n123 = Open/Create/Replace File(file path (use dialog)=w145) -> (refnum out=w162:refnum<file>, error out=w161:errorcluster)  [unwired: 1 in, 5 out]
        n124 = Open/Create/Replace File(file path (use dialog)=w144) -> (refnum out=w156:refnum<file>, error out=w155:errorcluster)  [unwired: 1 in, 5 out]
        n125 = Set File Position(offset (in bytes) (0)=i64 0 ("Offset (in Byte) (0)"), refnum=w162, from (0:start)=enum16{"start", "end", "current"}."end" ("Von (0:Start)"), error in=w161) -> (refnum out=w160:refnum<file>, error out=w158:errorcluster)
        n126 = Set File Position(offset (in bytes) (0)=i64 0 ("Offset (in Byte) (0)"), refnum=w156, from (0:start)=enum16{"start", "end", "current"}."end" ("Von (0:Start)"), error in=w155) -> (refnum out=w154:refnum<file>, error out=w152:errorcluster)
        n127 = Write to Text File(file (use dialog)=w160, text=w150, error in=w158) -> (refnum out=w159:refnum<file>, error out=w157:errorcluster)  [unwired: 1 in, 1 out]
        n128 = Write to Text File(file (use dialog)=w154, text=w150, error in=w152) -> (refnum out=w153:refnum<file>, error out=w151:errorcluster)  [unwired: 1 in, 1 out]
        n129 = Close File(refnum=w159, error in=w157) -> ()  [unwired: 2 out]
        n130 = Close File(refnum=w153, error in=w151) -> ()  [unwired: 2 out]
        n131 = call <vilib>:"DAQmx Stop Task.vi"("task/channels in"=w237, "error in"=w236) -> ("task out"=w244:refnum<k21>, "error out"=w243:errorcluster)  [unwired: 12 in]
        n132 = call <vilib>:"DAQmx Clear Task.vi"("task in"=w244, "error in"=w243) -> ("error out"=w242:errorcluster)  [unwired: 13 in]
        n133 = call <vilib>:"Simple Error Handler.vi"("error in (no error)"=w242) -> ()  [unwired: 4 in, 5 out]
        n134 = call <vilib>:"DAQmx Stop Task.vi"("task/channels in"=w239, "error in"=w238) -> ("task out"=w247:refnum<k21>, "error out"=w246:errorcluster)  [unwired: 12 in]
        n135 = call <vilib>:"DAQmx Clear Task.vi"("task in"=w247, "error in"=w246) -> ("error out"=w245:errorcluster)  [unwired: 13 in]
        n136 = call <vilib>:"Simple Error Handler.vi"("error in (no error)"=w245) -> ()  [unwired: 4 in, 5 out]
        n137 = call <vilib>:"DAQmx Stop Task.vi"("task/channels in"=w241, "error in"=w240) -> ("task out"=w250:refnum<k21>, "error out"=w249:errorcluster)  [unwired: 12 in]
        n138 = call <vilib>:"DAQmx Clear Task.vi"("task in"=w250, "error in"=w249) -> ("error out"=w248:errorcluster)  [unwired: 13 in]
        n139 = call <vilib>:"Simple Error Handler.vi"("error in (no error)"=w248) -> ()  [unwired: 4 in, 5 out]
        n140 = call <vilib>:"DAQmx Stop Task.vi"("task/channels in"=w266, "error in"=w267) -> ("task out"=w275:refnum<k21>, "error out"=w274:errorcluster)  [unwired: 12 in]
        n141 = call <vilib>:"DAQmx Clear Task.vi"("task in"=w275, "error in"=w274) -> ("error out"=w273:errorcluster)  [unwired: 13 in]
        n142 = call <vilib>:"Simple Error Handler.vi"("error in (no error)"=w273) -> ()  [unwired: 4 in, 5 out]
        n143 = call <vilib>:"DAQmx Stop Task.vi"("task/channels in"=w281, "error in"=w277) -> ("task out"=w280:refnum<k21>, "error out"=w279:errorcluster)  [unwired: 12 in]
        n144 = call <vilib>:"DAQmx Clear Task.vi"("task in"=w280, "error in"=w279) -> ("error out"=w278:errorcluster)  [unwired: 13 in]
        n145 = call <vilib>:"Simple Error Handler.vi"("error in (no error)"=w278) -> ()  [unwired: 4 in, 5 out]
      }
      n146 = Two Button Dialog(message="Failure?\nDiscard Measurement?" ("String"), 1:"NO" ("String"), 2:"Yes" ("String")) -> (T button?=w105:bool)
      n147 = case shown="False" w105 {
        tunnel: w110 -> [_ w114]
        tunnel: w109 -> [_ w113]
        frame False {
        }
        frame True {
          w112 = "#FEHLER#" ("String")
          n148 = Open/Create/Replace File(file path (use dialog)=w114) -> (refnum out=w130:refnum<file>, error out=w129:errorcluster)  [unwired: 1 in, 5 out]
          n149 = Open/Create/Replace File(file path (use dialog)=w113) -> (refnum out=w124:refnum<file>, error out=w123:errorcluster)  [unwired: 1 in, 5 out]
          n150 = Set File Position(offset (in bytes) (0)=i64 0 ("Offset (in Byte) (0)"), refnum=w130, from (0:start)=enum16{"start", "end", "current"}."start" ("Von (0:Start)"), error in=w129) -> (refnum out=w128:refnum<file>, error out=w126:errorcluster)
          n151 = Set File Position(offset (in bytes) (0)=i64 0 ("Offset (in Byte) (0)"), refnum=w124, from (0:start)=enum16{"start", "end", "current"}."start" ("Von (0:Start)"), error in=w123) -> (refnum out=w122:refnum<file>, error out=w120:errorcluster)
          n152 = Write to Text File(file (use dialog)=w128, text=w112, error in=w126) -> (refnum out=w127:refnum<file>, error out=w125:errorcluster)  [unwired: 1 in, 1 out]
          n153 = Write to Text File(file (use dialog)=w122, text=w112, error in=w120) -> (refnum out=w121:refnum<file>, error out=w119:errorcluster)  [unwired: 1 in, 1 out]
          n154 = Close File(refnum=w127, error in=w125) -> ()  [unwired: 2 out]
          n155 = Close File(refnum=w121, error in=w119) -> ()  [unwired: 2 out]
        }
      }
    }
    frame Default {
      # "This diagram executes if the enum value is anything other than what is specified in the other cases of this case structure."
    }
  }
